vi "Is_TestDataInSpec-.vi"(4 "Row":i32, 6 "量测项目":string[][](array[string]), 7 "相机量测结果":dbl[](array[numeric])) -> (0 "修正后相机量测结果":dbl[](array[numeric]), 1 "在规格内 数组":bool[](array[boolean]), 2 "进位舍位后值":dbl[](array[numeric]), 3 "在规格内":bool)   [LabVIEW 2014]
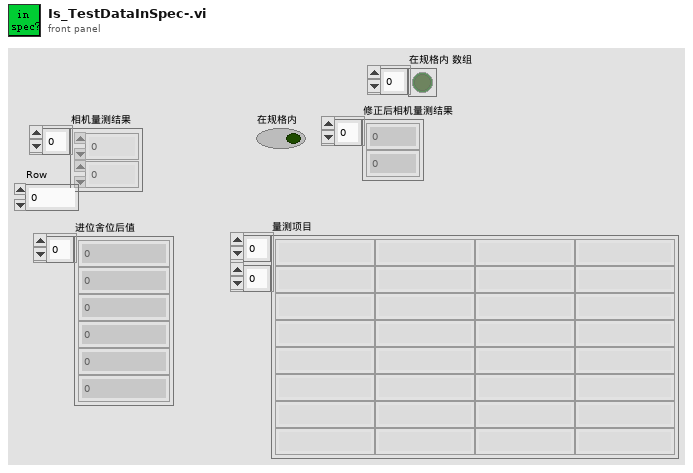
[diagram p1: front panel]
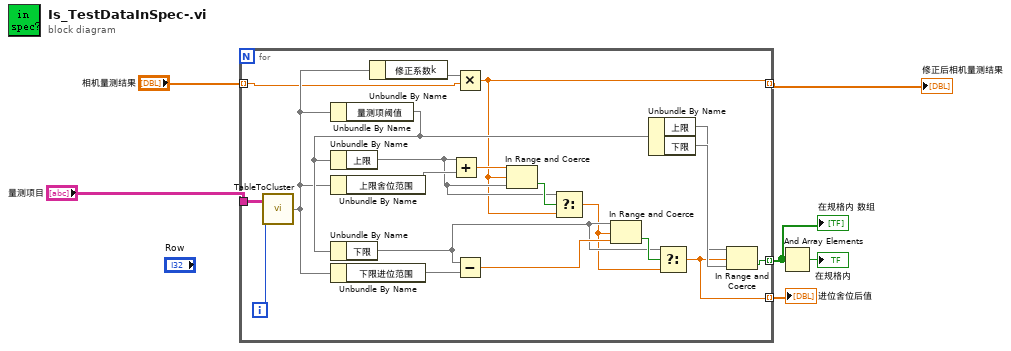
[diagram p0: block diagram]
diagram:
  n1 = for {
    tunnel: "相机量测结果" -> [w8] mode=indexing
    tunnel: [w26] -> w5 mode=indexing
    tunnel: "量测项目" -> [w25]
    tunnel: [w14] -> w2 mode=indexing
    tunnel: [w7] -> w1 mode=indexing
    i -> [w11]
    n2 = call "TableToCluster.vi"(1:w11, 2:w25) -> (0:w10)
    n3 = Unbundle By Name(w10) -> ("量测项阈值"=w13)
    n4 = Unbundle By Name(w13) -> ("上限"=w12)
    n5 = Unbundle By Name(w10) -> ("上限舍位范围"=w24)
    n6 = Unbundle By Name(w13) -> ("下限"=w17)
    n7 = Unbundle By Name(w10) -> ("下限进位范围"=w16)
    n8 = Unbundle By Name(w10) -> ("修正系数k"=w9)
    n9 = Add(x=w12, y=w24) -> (x+y=w23:dbl)
    n10 = Multiply(x=w9, y=w8) -> (x*y=w7:dbl)
    n11 = Subtract(x=w17, y=w16) -> (x-y=w20:dbl)
    n12 = In Range and Coerce(upper limit=w23, x=w7, lower limit=w12) -> (In Range?=w22:bool)  [unwired: 1 out]
    n13 = Select(t=w12, s=w22, f=w7) -> (s? t:f=w15:dbl)
    n14 = In Range and Coerce(upper limit=w17, x=w15, lower limit=w20) -> (In Range?=w21:bool)  [unwired: 1 out]
    n15 = Unbundle By Name(w13) -> ("上限"=w18, "下限"=w19)
    n16 = Select(t=w17, s=w21, f=w15) -> (s? t:f=w14:dbl)
    n17 = In Range and Coerce(upper limit=w18, x=w14, lower limit=w19) -> (In Range?=w26:bool)  [unwired: 1 out]
  }
  "进位舍位后值" <- w2
  "在规格内 数组" <- w5
  "修正后相机量测结果" <- w1
  n18 = And Array Elements(Boolean array=w5) -> (logical AND=→"在规格内":bool)
